vi "IIR Comb Filter Design.vi"() -> ()   [LabVIEW 2023]
doc: "Demonstrates how to use the DFD IIR Comb Design VI to design different types of comb filters with different sets of parameters.\n\nComplete the following steps to use this VI.\n1) Run the VI.\n2) Click <B>By N and Bandwidth</B> to set the design method, and change <B>N</B>, <B>Bandwidth</B>, and <B>Ab</B>.\n3) Observe the magnitude response of the designed filter.\n4) Change the <B>Filter Type</B> and observe the magnitude response.\n5) Click <B>By f0 and Bandwidth</B> to set the design method, and change <B>f0</B>, <B>fs</B>, <B>Bandwidth</B>, and <B>Ab</B>. \n6) Observe the magnitude response of the designed filter.\n7) Change the <B>Filter Type</B> and observe the magnitude response.\n8) Click the <B>STOP</B> button to stop this VI."
uses:
  <vilib>/addons/Digital Filter Design/Design.llb/DFD IIR Comb Design by N and BW.vi
  <vilib>/addons/Digital Filter Design/Design.llb/DFD IIR Comb Design by f and BW.vi
  <vilib>/addons/Digital Filter Design/Analysis.llb/DFD Plot Freq Response (Linear-Spaced).vi
  <vilib>/addons/Digital Filter Design/NI_DigFilterLicensed.lvlib
panel:
  in  "Sampling Frequency [Hz]":dbl=600.0 format="%.2f"
  in  "Tab Control":T1(tab)=enum."By f0 and Bandwidth"
  in  "N":i32=10
  in  "f0 [Hz]":dbl=60.0 format="%.2f"
  in  "Filter Type":T2(ring)
  in  "Ab [dB]":dbl=3.010299956639812 format="%#.6g"
  in  "Bandwidth [Hz]":dbl=0.6 format="%#_2f"
  in  "stop":bool
  out "Error Message":string
  out "Magnitude Response":cluster{"f0":dbl, "df":dbl, "values":dbl[]}[](graph)
  # "Select Help>>Show Context Help and move the cursor over the VI icon for more information."
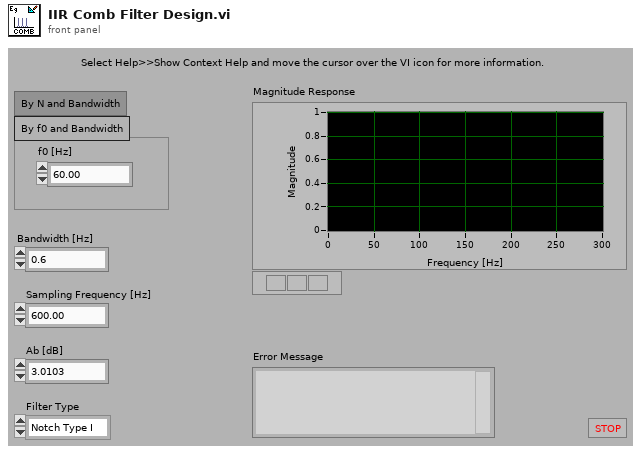
[diagram p1: front panel]
types:
  T1 = enum32{"By N and Bandwidth", "By f0 and Bandwidth"}
  T2 = enum16{"Notch Type I", "Notch Type II", "Peak Type I", "Peak Type II"}
  T3 = typedef "NI_DigFilterLicensed.lvlib/DFD Filter Obj.ctl" = cluster{"mSRate_Fs":dbl, "mSRate_Version":string, "mSRate_Comments":string, "mSRate_OrgCoef":T4, "mSRate_CurCoef":T4, "mSRate_Quantized?":bool, "mSRate_QCoef":T4, "mSRate_QSettings":T6[], "mSRate_Order":i32, "mSRate_Scaling":cluster{"mSRate_ScaleByPowerOf2?":bool, "mSRate_ScaleType":T8}}
  T4 = typedef "NI_DigFilterLicensed.lvlib/DFD Filter Coef.ctl" = cluster{"type":T5, "gain":dbl, "coef a (k)":dbl[], "coef b (v)":dbl[]}
  T5 = typedef "NI_DigFilterLicensed.lvlib/DFD Filter Structure Type Selector.ctl" = enum16{"Undefined", "FIR Direct Form", "FIR Direct Form Transposed", "FIR Symmetric", "FIR Antisymmetric", "IIR Direct Form I", "IIR Direct Form I Transposed", "IIR Direct Form II", "IIR Direct Form II Transposed", "IIR Cascaded Second Order Sections Form I", "IIR Cascaded Second Order Sections Form I Transposed", "IIR Cascaded Second Order Sections Form II", "IIR Cascaded Second Order Sections Form II Transposed", "Lattice Allpass (basic sections)", "Lattice Allpass (one multiplier sections)", "Lattice Allpass (normalized sections)", "Lattice AR (basic sections)", "Lattice AR (one multiplier sections)", "Lattice AR (normalized sections)", "Lattice MA (minimum phase)", "Lattice MA (maximum phase)", "Lattice ARMA (basic sections)", "Lattice ARMA (one multiplier sections)", "Lattice ARMA (normalized sections)"}
  T6 = typedef "NI_DigFilterLicensed.lvlib/dfd_Internal Quantization Settings.ctl" = cluster{"source":T7, "wl":i16, "iwl":i16, "overflow mode":enum16{"Saturation", "Wrap"}, "rounding mode":enum16{"Nearest", "Truncation"}, "signed?":bool}
  T7 = typedef "NI_DigFilterLicensed.lvlib/dfd_Internal Quantization Srcs.ctl" = u16
  T8 = typedef "NI_DigFilterLicensed.lvlib/DFD Coef Norm Type.ctl" = enum16{"No Norm", "Time Domain 1-Norm", "Time Domain 2-Norm", "Time Domain Inf-Norm"}
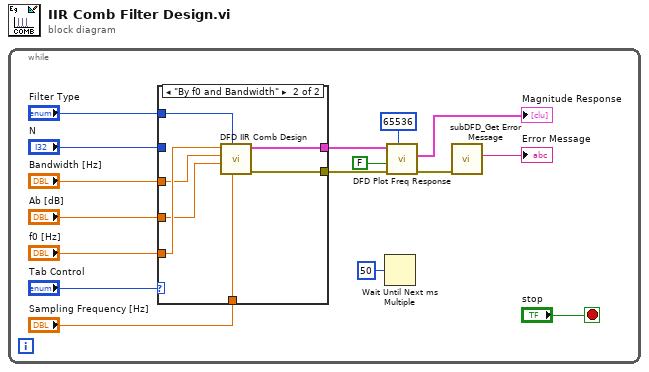
[diagram p0: block diagram]
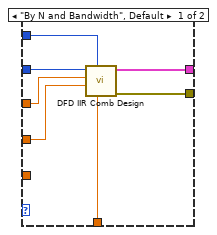
[diagram p2: hidden frame]
diagram:
  n1 = while {
    stop <- "stop" stop-if-true
    n2 = case shown="\"By f0 and Bandwidth\"" "Tab Control" {
      tunnel: [w23 w30] -> w15
      tunnel: [w22 w29] -> w14
      tunnel: "N" -> [w21 _]
      tunnel: "Bandwidth [Hz]" -> [w20 w27]
      tunnel: "Ab [dB]" -> [w19 w26]
      tunnel: "f0 [Hz]" -> [_ w28]
      tunnel: "Sampling Frequency [Hz]" -> [w17 w25]
      tunnel: "Filter Type" -> [w18 w24]
      frame "By N and Bandwidth", Default {
        n3 = call-poly <vilib>:"DFD IIR Comb Design.vi"("fs [Hz]"=w17, "filter type"=w18, "Ab [dB]"=w19, "Df [Hz]"=w20, "# notches/peaks"=w21) -> ("error out"=w22:errorcluster, "filter out"=w23:T3)  [unwired: 1 in, 4 out]
      }
      frame "By f0 and Bandwidth" {
        n4 = call-poly <vilib>:"DFD IIR Comb Design.vi"("fs [Hz]"=w25, "filter type"=w24, "Ab [dB]"=w26, "Df [Hz]"=w27, "f0 [Hz]"=w28) -> ("error out"=w29:errorcluster, "filter out"=w30:T3)  [unwired: 1 in, 4 out]
      }
    }
    n5 = Wait Until Next ms Multiple(millisecond multiple=u32 50) -> ()  [unwired: 1 out]
    n6 = call-poly <vilib>:"DFD Plot Freq Response.vi"("# freq bins"=65536 ("# freq bins (auto)"), "error in (no error)"=w14, "dB on? (T)"=FALSE, "filter in"=w15) -> ("error out"=w9:errorcluster, "magnitude response"=→"Magnitude Response":cluster{"f0":dbl, "df":dbl, "values":dbl[]}[])  [unwired: 4 in, 2 out]
    n7 = call <vilib>:"subDFD_Get Error Message.vi"("error in (no error)"=w9) -> ("Error Message"=→"Error Message":string)  [unwired: 10 out]
  }
